vi "Tester.vi"() -> ()   [LabVIEW 2020]
uses:
  CLD3 FGV Mode.ctl
panel:
  out "Has Time Elapsed":bool
  in  "stop":bool
  out "Elapsed Time (s.ss)":dbl
  out "Error Out":errorcluster
  in  "Timer Mode":T1
  in  "Time Target (s)":dbl=4.0
  in  "Error In":errorcluster
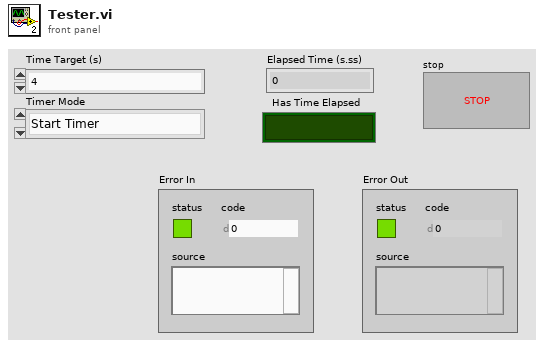
[diagram p1: front panel]
types:
  T1 = typedef "CLD3 FGV Mode.ctl" = enum16{"Start Timer", "Read Time", "Pause", "Resume"}
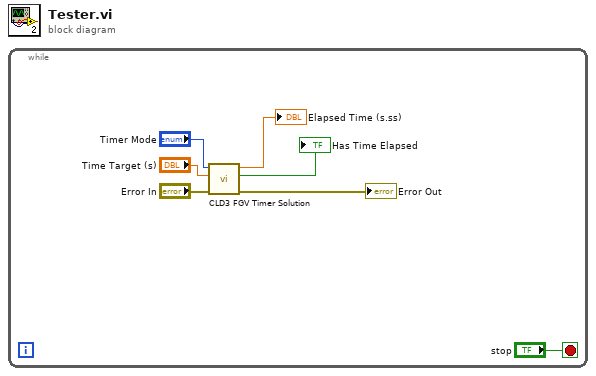
[diagram p0: block diagram]
diagram:
  n1 = while {
    stop <- "stop" stop-if-true
    n2 = call "CLD3 FGV Timer Solution.vi"("Error In"="Error In", "Time Target (s)"="Time Target (s)", "Timer Mode"="Timer Mode") -> ("Error Out"=→"Error Out":errorcluster, "Has Time Elapsed"=→"Has Time Elapsed":bool, "Elapsed Time (s.ss)"=→"Elapsed Time (s.ss)":dbl)  [unwired: 6 in]
  }
